vi "Display Window.vi"(0 "Document in":refnum<class "Document.lvclass">, 11 "error in (no error)":errorcluster) -> (4 "Document out":refnum<class "Document.lvclass">, 15 "error out":errorcluster)   [LabVIEW 2016, in "Document.lvclass"]
uses:
  Document.lvclass
  Document.lvclass/Document.ctl
  user32.dll
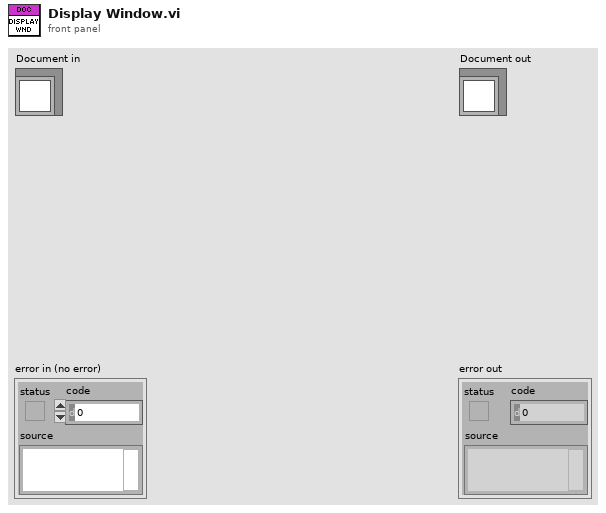
[diagram p1: front panel]
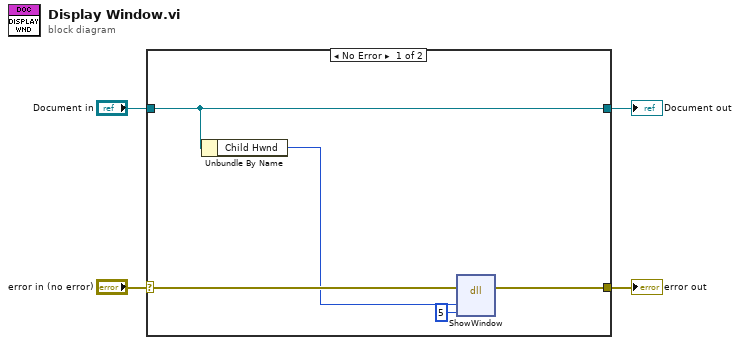
[diagram p0: block diagram]
diagram:
  n1 = case shown="No Error" "error in (no error)" {
    selector: "error in (no error)" -> [w8 w11]
    tunnel: [w7 w11] -> w3
    tunnel: [w6 w10] -> w1
    tunnel: "Document in" -> [w6 w10]
    frame No Error {
      n2 = Unbundle By Name(w6) -> ("Child Hwnd"=w5:u32)
      n3 = dll-call lib="user32.dll" fn="ShowWindow"(error in=w8, "hwnd"=w5, "nCmdShow"=u32 5) -> (error out=w7:errorcluster)  [unwired: 5 in, 1 out]
    }
    frame Error {
    }
  }
  "error out" <- w3
  "Document out" <- w1
